vi "Raster Parameters2.vi"(0 "Pixels":i32=700, 2 "X Offset [um]":ext, 5 "Lines/s":dbl=20.0, 9 "Scan Size [um]":dbl=10.0, 11 "error in (no error)":errorcluster, 13 "Y Offset [um]":ext) -> (1 "X Step Size":fxp<+,30,1>=0.002616431564092636, 3 "Half X Scan Size":fxp<+,24,3>=0.9157509803771973, 4 "X Steps":u32=699, 6 "Y Steps":u64=978600, 12 "Y Step Size":fxp<+,30,1>=1.3057142496109009e-06, 14 "Half Y Scan Size":fxp<+,24,3>=0.6385698318481445, 15 "error out":errorcluster)   [LabVIEW 2017]
panel:
  out "Sample Rate [us]":dbl=35.0
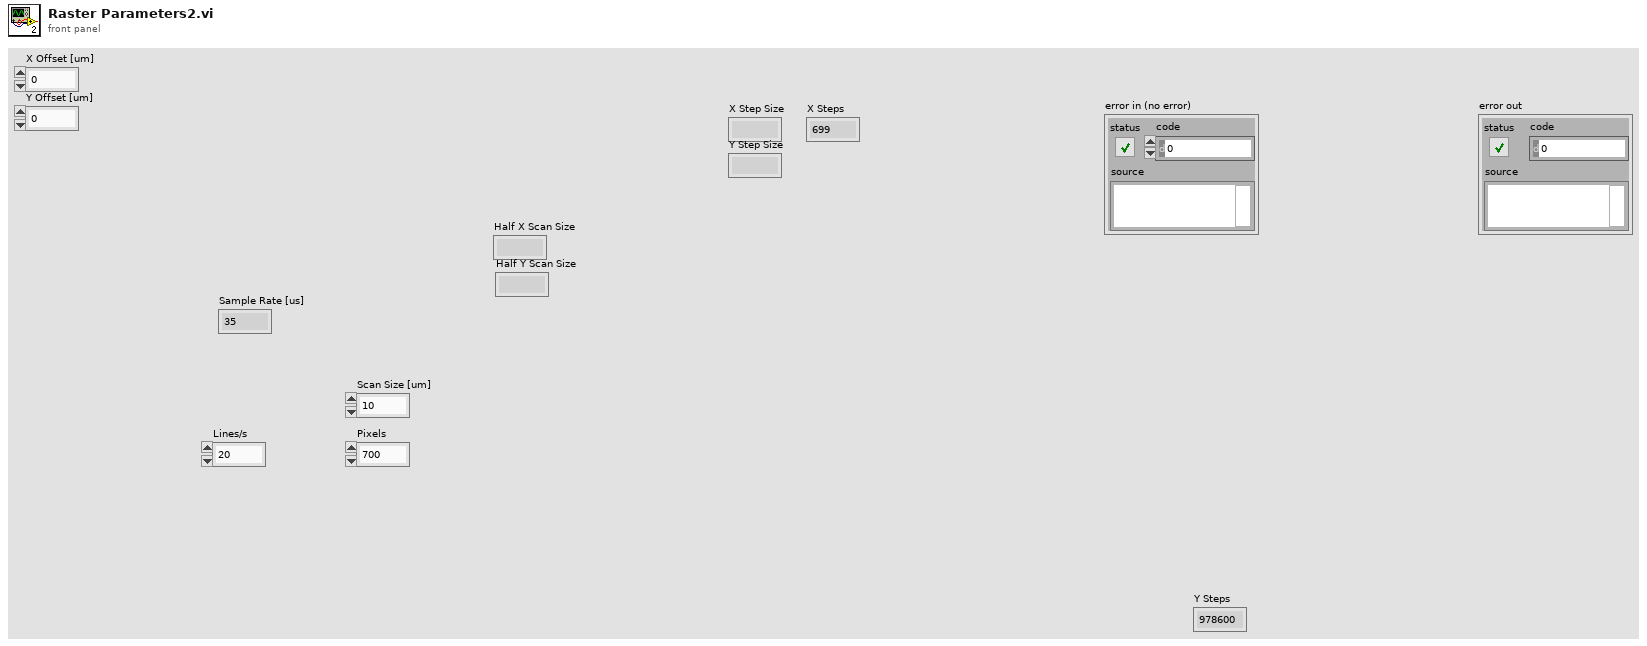
[diagram p1: front panel]
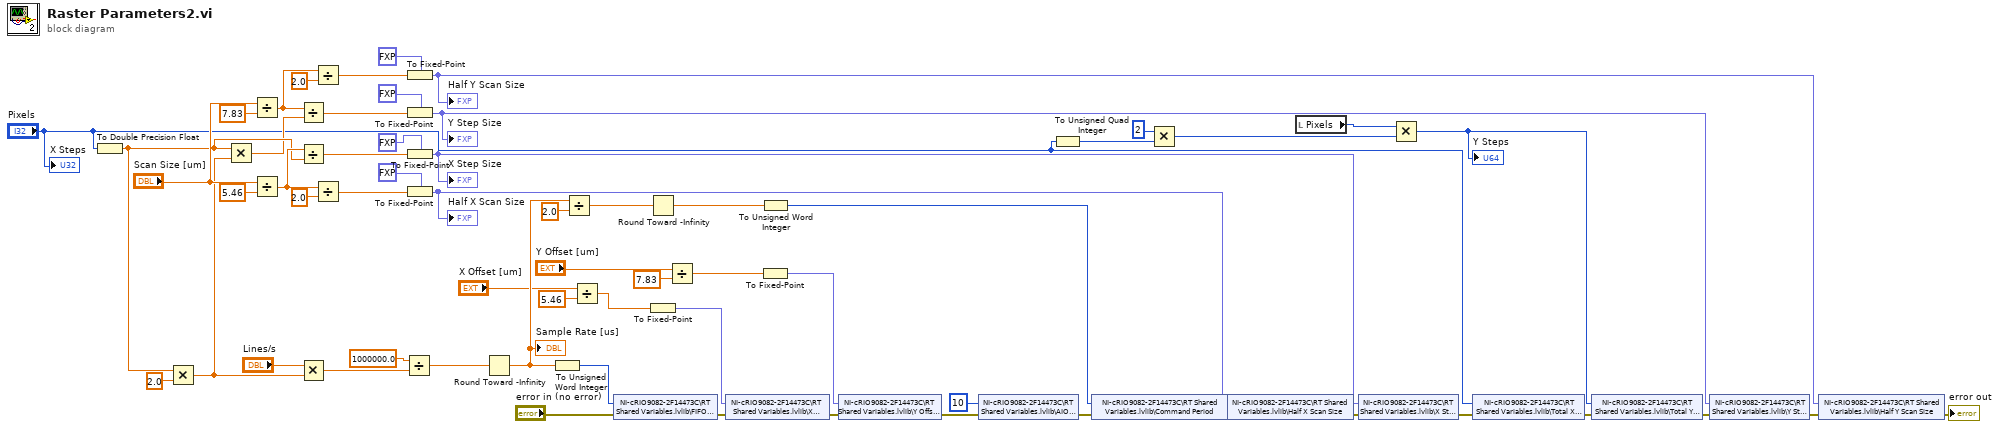
[diagram p0: block diagram]
diagram:
  n1 = To Double Precision Float(number="Pixels") -> (double precision float=w16:dbl)
  n2 = Multiply(x=w16, y=2.0) -> (x*y=w17:dbl)
  n3 = Multiply(x=w16, y=w17) -> (x*y=w14:dbl)
  n4 = Divide(x="Scan Size [um]", y=7.83) -> (x/y=w15:dbl)
  n5 = Divide(x="Scan Size [um]", y=5.46) -> (x/y=w59:dbl)
  n6 = Divide(x=w15, y=w14) -> (x/y=w13:dbl)
  n7 = Divide(x=w59, y=w16) -> (x/y=w18:dbl)
  n8 = Multiply(x="Lines/s", y=w17) -> (x*y=w45:dbl)
  n9 = Divide(x=w15, y=2.0) -> (x/y=w52:dbl)
  n10 = Divide(x=w59, y=2.0) -> (x/y=w55:dbl)
  n11 = Divide(x=1000000.0, y=w45) -> (x/y=w47:dbl)
  n12 = To Fixed-Point(fixed-point type=fxp<+,24,3> 0.0 ("Half X Scan Size"), number=w52) -> (fixed-point=w32:fxp<+,24,3>)
  "Half Y Scan Size" <- w32
  n13 = To Fixed-Point(fixed-point type=fxp<+,30,1> 0.0 ("X Step Size"), number=w13) -> (fixed-point=w31:fxp<+,30,1>)
  "Y Step Size" <- w31
  n14 = To Fixed-Point(fixed-point type=fxp<+,30,1> 0.0 ("X Step Size"), number=w18) -> (fixed-point=w36:fxp<+,30,1>)
  "X Step Size" <- w36
  n15 = To Fixed-Point(fixed-point type=fxp<+,24,3> 0.0 ("Half X Scan Size"), number=w55) -> (fixed-point=w37:fxp<+,24,3>)
  "Half X Scan Size" <- w37
  n16 = Round Toward -Infinity(1:w47) -> (0:w38:dbl)
  "Sample Rate [us]" <- w38
  n17 = To Unsigned Word Integer(number=w38) -> (unsigned 16bit integer=w21:u16)
  n18 = Divide(x=w38, y=2.0) -> (x/y=w41:dbl)
  n19 = Divide(x="X Offset [um]", y=5.46) -> (x/y=w7:ext)
  n20 = shared-variable "NI-cRIO9082-2F14473C\\RT Shared Variables.lvlib\\FIFO Period"(w21, error in="error in (no error)") -> (error out=w3:errorcluster)
  n21 = Round Toward -Infinity(1:w41) -> (0:w40:dbl)
  n22 = To Fixed-Point(number=w7) -> (fixed-point=w11:fxp<+/-,33,5>)  [unwired: 1 in]
  n23 = Divide(x="Y Offset [um]", y=7.83) -> (x/y=w4:ext)
  n24 = shared-variable "NI-cRIO9082-2F14473C\\RT Shared Variables.lvlib\\X Offset [V]"(w11, error in=w3) -> (error out=w2:errorcluster)
  n25 = To Unsigned Word Integer(number=w40) -> (unsigned 16bit integer=w20:u16)
  n26 = To Fixed-Point(number=w4) -> (fixed-point=w10:fxp<+/-,33,5>)  [unwired: 1 in]
  n27 = shared-variable "NI-cRIO9082-2F14473C\\RT Shared Variables.lvlib\\Y Offset [V]"(w10, error in=w2) -> (error out=w1:errorcluster)
  n28 = shared-variable "NI-cRIO9082-2F14473C\\RT Shared Variables.lvlib\\AIO Period"(u16 10 ("AIO Period"), error in=w1) -> (error out=w23:errorcluster)
  n29 = To Unsigned Quad Integer(1:"Pixels") -> (0:w35:u64)
  n30 = shared-variable "NI-cRIO9082-2F14473C\\RT Shared Variables.lvlib\\Command Period"(w20, error in=w23) -> (error out=w22:errorcluster)
  n31 = Multiply(x=u64 2, y=w35) -> (x*y=w56:u64)
  n32 = shared-variable "NI-cRIO9082-2F14473C\\RT Shared Variables.lvlib\\Half X Scan Size"(w37, error in=w22) -> (error out=w30:errorcluster)
  n33 = local read "Pixels"() -> (w57:i32)
  n34 = shared-variable "NI-cRIO9082-2F14473C\\RT Shared Variables.lvlib\\X Step Size"(w36, error in=w30) -> (error out=w29:errorcluster)
  n35 = Multiply(x=w57, y=w56) -> (x*y=w33:u64)
  "Y Steps" <- w33
  n36 = shared-variable "NI-cRIO9082-2F14473C\\RT Shared Variables.lvlib\\Total X Steps"("Pixels", error in=w29) -> (error out=w28:errorcluster)
  n37 = shared-variable "NI-cRIO9082-2F14473C\\RT Shared Variables.lvlib\\Total Y Steps"(w33, error in=w28) -> (error out=w27:errorcluster)
  n38 = shared-variable "NI-cRIO9082-2F14473C\\RT Shared Variables.lvlib\\Y Step Size"(w31, error in=w27) -> (error out=w26:errorcluster)
  n39 = shared-variable "NI-cRIO9082-2F14473C\\RT Shared Variables.lvlib\\Half Y Scan Size"(w32, error in=w26) -> (error out=→"error out":errorcluster)
  "X Steps" <- "Pixels"
